vi "Create Message.vi"(0 "CMD String":string, 1 "Type of Message":T2, 2 "Timeout in ms (-1)":i32, 5 "Sender Name":string, 7 "Recipent Name":string, 9 "Data":variant, 11 "Error In":errorcluster, 12 "Return State":string) -> (4 "Wait Notifier":refnum<notifier>, 8 "Message":T1, 15 "Error Out":errorcluster)   [LabVIEW 2023, in "Message Handler.lvclass"]
doc: "Composes full message based on inputs provided."
uses:
  Message Handler.lvclass
  Public/Ctrls/Type of Message.ctl
  Interfaces/ICanCommunicate/Message.ctl
  Message Handler.lvclass/Message Handler.ctl
  Interfaces/ICanCommunicate/ICanCommunicate.lvclass
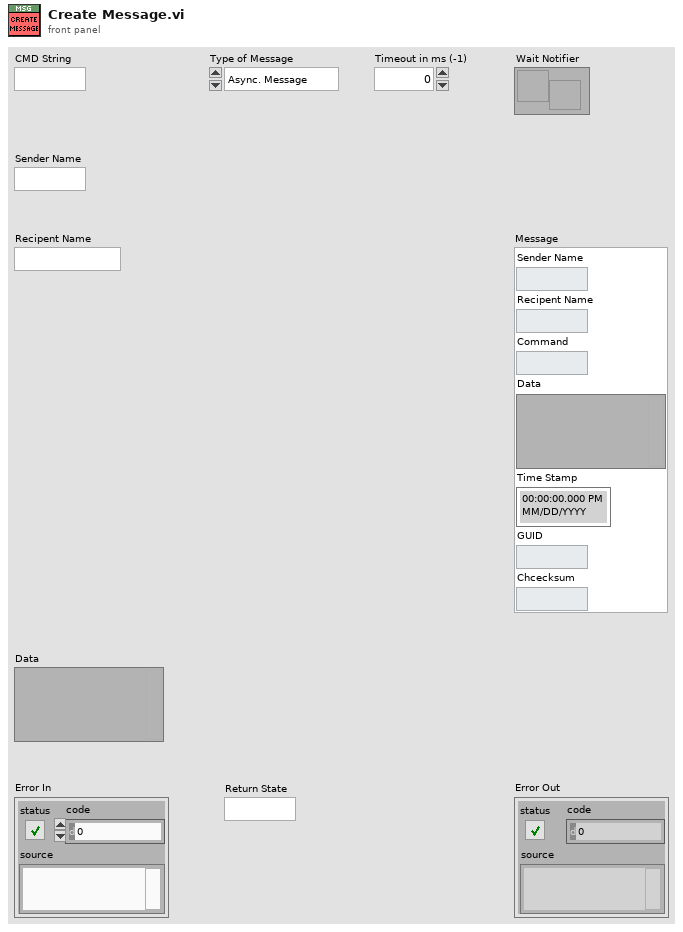
[diagram p1: front panel]
types:
  T1 = typedef "ICanCommunicate.lvclass/Message.ctl" = cluster{"Sender Name":string, "Recipent Name":string, "Command":string, "Data":variant, "Time Stamp":timestamp, "GUID":string, "Chcecksum":string}
  T2 = typedef "Message Handler.lvclass/Type of Message.ctl" = enum16{"Async. Message", "Async. Data Request", "Sync. Data Request"}
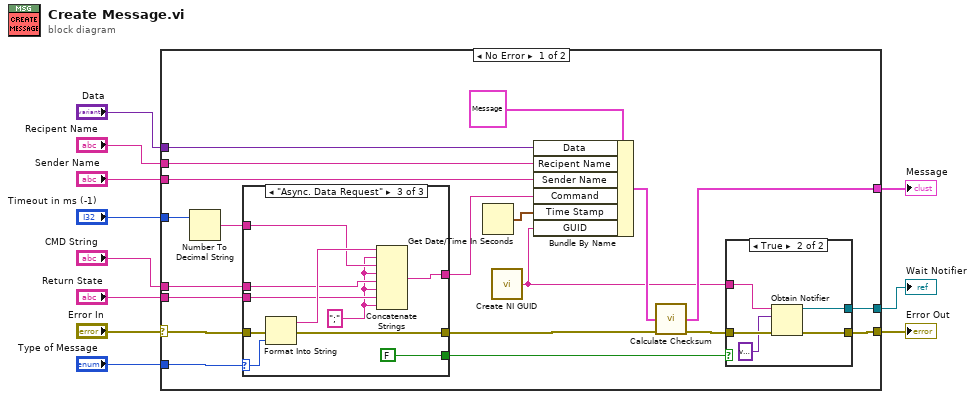
[diagram p0: block diagram]
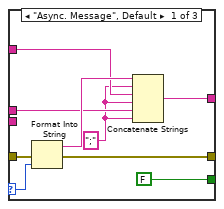
[diagram p2: hidden frame]
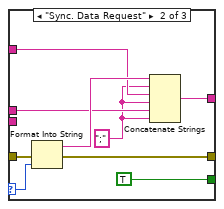
[diagram p3: hidden frame]
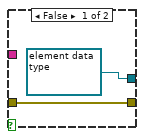
[diagram p4: hidden frame]
diagram:
  n1 = case shown="No Error" "Error In" {
    selector: "Error In" -> [w30 w67]
    tunnel: "Data" -> [w18 _]
    tunnel: "Recipent Name" -> [w17 _]
    tunnel: [w23 _] -> w9
    tunnel: "Type of Message" -> [w31 _]
    tunnel: "Sender Name" -> [w16 _]
    tunnel: "CMD String" -> [w29 _]
    tunnel: "Return State" -> [w28 _]
    tunnel: [w24 w67] -> w3
    tunnel: [w22 _] -> w2
    tunnel: "Timeout in ms (-1)" -> [w15 _]
    frame No Error {
      n2 = Number To Decimal String(number=w15) -> (decimal integer string=w14:string)  [unwired: 1 in]
      n3 = case shown="\"Async. Data Request\"" w31 {
        selector: w31 -> [w40 w49 w59]
        tunnel: w14 -> [w37 w46 w56]
        tunnel: w30 -> [w39 w48 w58]
        tunnel: w29 -> [w36 w45 w55]
        tunnel: w28 -> [_ _ w51]
        tunnel: [w35 w44 w54] -> w27
        tunnel: [FALSE TRUE FALSE] -> w25
        tunnel: [w33 w41 w52] -> w20
        frame "Async. Message", Default {
          w32 = ";"
          n4 = Format Into String(error in=w39, w40) -> (resulting string=w38:string, error out=w35:errorcluster)  [unwired: 2 in]
          n5 = Concatenate Strings(w38, w32, w37, w32, w36, w32) -> (w33:string)
        }
        frame "Sync. Data Request" {
          w42 = ";"
          n6 = Format Into String(error in=w48, w49) -> (resulting string=w47:string, error out=w44:errorcluster)  [unwired: 2 in]
          n7 = Concatenate Strings(w47, w42, w46, w42, w45, w42) -> (w41:string)
        }
        frame "Async. Data Request" {
          w50 = ";"
          n8 = Format Into String(error in=w58, w59) -> (resulting string=w57:string, error out=w54:errorcluster)  [unwired: 2 in]
          n9 = Concatenate Strings(w57, w50, w56, w50, w55, w50, w51, w50) -> (w52:string)
        }
      }
      n10 = Get Date/Time In Seconds() -> (seconds since 1Jan1904=w13:timestamp)
      n11 = call <vilib>:"Create NI GUID.vi"() -> ("NI GUID"=w12:string)
      n12 = Bundle By Name(cluster=T1 {"Sender Name"="", "Recipent Name"="", "Command"="", "Data"=variant, "Time Stamp"=timestamp(0 s since 1904-01-01), "GUID"="", "Chcecksum"=""} ("Message"), "Data"=w18, "Recipent Name"=w17, "Sender Name"=w16, "Command"=w20, "Time Stamp"=w13, "GUID"=w12) -> (w19:T1)
      n13 = call "Calculate Checksum.vi"("Message In"=w19, "Error In"=w27) -> ("Message Out"=w23:T1, "Error Out"=w26:errorcluster)  [unwired: 11 in, 1 out]
      n14 = case shown="True" w25 {
        tunnel: w26 -> [w61 w66]
        tunnel: w12 -> [_ w65]
        tunnel: [w61 w63] -> w24
        tunnel: [refnum<notifier> refnum ("notifier out") w62] -> w22
        frame False {
        }
        frame True {
          n15 = Obtain Notifier(name (unnamed)=w65, notification data type=variant ("element data type"), error in (no error)=w66) -> (notifier out=w62:refnum<notifier>, error out=w63:errorcluster)  [unwired: 1 in, 1 out]
        }
      }
    }
    frame Error {
      # "#TO_DO error handle?"
    }
  }
  "Message" <- w9
  "Error Out" <- w3
  "Wait Notifier" <- w2
